vi "Read Dequeuer.vi"(11 "Message Queue":refnum<class "Message Queue.lvclass">) -> (2 "Message Dequeuer":refnum<class "Message Dequeuer.lvclass">)   [LabVIEW 2020, in "Actor Framework.lvlib" / "Message Queue.lvclass"]
doc: "<p>(<strong>Filename</strong>: <span class=\"dnl\">Actor Framework.lvlib:Message Queue.lvclass:Read Dequeuer.vi</span>)</p>\n\n<p>Extracts the reference needed to read messages from the top-level actor.</p>\n\n<p>Use the <a href=\"nihelplauncher://docs/csh?context=lvcore_lvcomm_af_obtain_message_q\">Obtain Message Queue</a> method to obtain the <strong>Message Queue</strong> input.</p>"
uses:
  Message Queue.lvclass
  Message Dequeuer/Message Dequeuer.lvclass
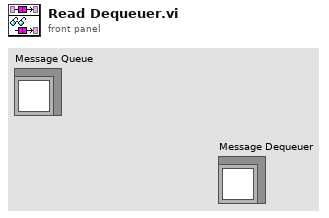
[diagram p1: front panel]
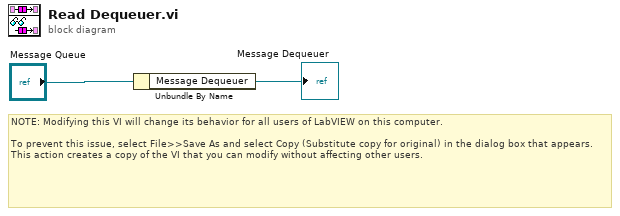
[diagram p0: block diagram]
diagram:
  # "NOTE: Modifying this VI will change its behavior for all users of LabVIEW on this computer.\n\nTo prevent this issue, select File>>Save As and select Copy (Substitute copy for original) in the dialog box that appears. This action creates a copy of the VI that you can modify without affecting other users."
  n1 = Unbundle By Name("Message Queue") -> ("Message Dequeuer"=→"Message Dequeuer":refnum<class "Message Dequeuer.lvclass">)
